vi "Get Serial Data.vi"(11 "SerialPortRef In":T1) -> (3 "SerialPortRef Out":T1)   [LabVIEW 2012]
uses:
  <vilib>/Rock Robotics/WPI/SerialPort/WPI_SerialPortRef.ctl
  Robot Global Data.vi
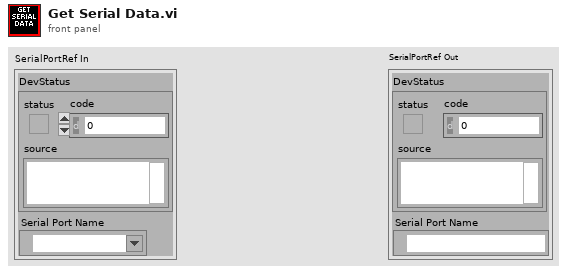
[diagram p1: front panel]
types:
  T1 = typedef "WPI_SerialPortRef.ctl" = cluster{"DevStatus":errorcluster, "Serial Port Name":refnum<visa-resource-name>}
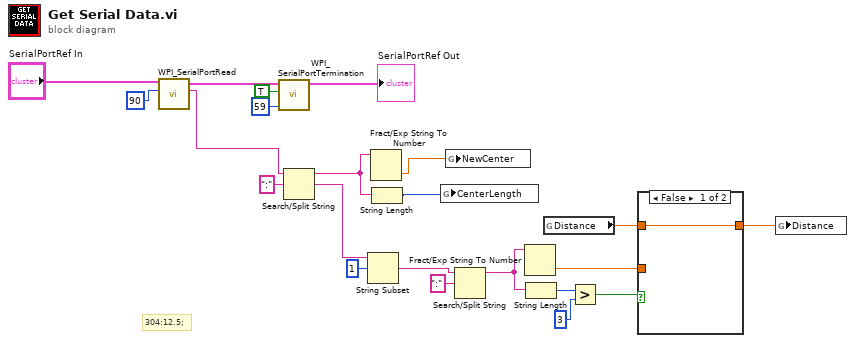
[diagram p0: block diagram]
diagram:
  # "304:12.5;"
  n1 = call <vilib>:"WPI_SerialPortRead.vi"("Num Bytes to Read"=u32 90, "SerialPortRef"="SerialPortRef In") -> ("Buffer"=w16:string, "SerialPortRef"=w22:T1)  [unwired: 7 in, 1 out]
  n2 = call <vilib>:"WPI_SerialPortTermination.vi"("Termination Char (0xA = '\\n' = LF)"=u8 59 ("Termination Char (0xA = '\\n' = LF)"), "Enable? (T)"=TRUE, "SerialPortRef"=w22) -> ("SerialPortRef"=→"SerialPortRef Out":T1)  [unwired: 7 in, 1 out]
  n3 = Search/Split String(string=w16, search string/char (-)=":") -> (substring before match=w17:string, match + rest of string=w14:string)  [unwired: 1 in, 1 out]
  n4 = String Subset(string=w14, offset (0)=1) -> (substring=w10:string)  [unwired: 1 in]
  n5 = Fract/Exp String To Number(string=w17) -> (number=w15:dbl)  [unwired: 3 in, 1 out]
  n6 = String Length(string=w17) -> (length=w12:i32)
  n7 = global write "Robot Global Data.vi" "CenterLength"(w12) -> ()
  n8 = global write "Robot Global Data.vi" "NewCenter"(w15) -> ()
  n9 = Search/Split String(string=w10, search string/char (-)=":") -> (substring before match=w9:string)  [unwired: 1 in, 2 out]
  n10 = Fract/Exp String To Number(string=w9) -> (number=w2:dbl)  [unwired: 3 in, 1 out]
  n11 = String Length(string=w9) -> (length=w7:i32)
  n12 = global read "Robot Global Data.vi" "Distance"() -> (w3:dbl)
  n13 = Greater?(x=w7, y=3) -> (0:w6:bool)
  n14 = case shown="False" w6 {
    tunnel: [w23 w24] -> w4
    tunnel: w3 -> [w23 _]
    tunnel: w2 -> [_ w24]
    frame False {
    }
    frame True {
    }
  }
  n15 = global write "Robot Global Data.vi" "Distance"(w4) -> ()
